vi "GantnerParameters.vi"() -> ()   [LabVIEW 2012]
uses:
  drivers/Gantner/Gantner-Instruments ISMBUS32.llb/ISMBUS_Module.ctl
  drivers/Gantner/Gantner-Instruments ISMBUS32.llb/ISMBUS_Channel.ctl
panel:
  in  "GantnerParameters":T3
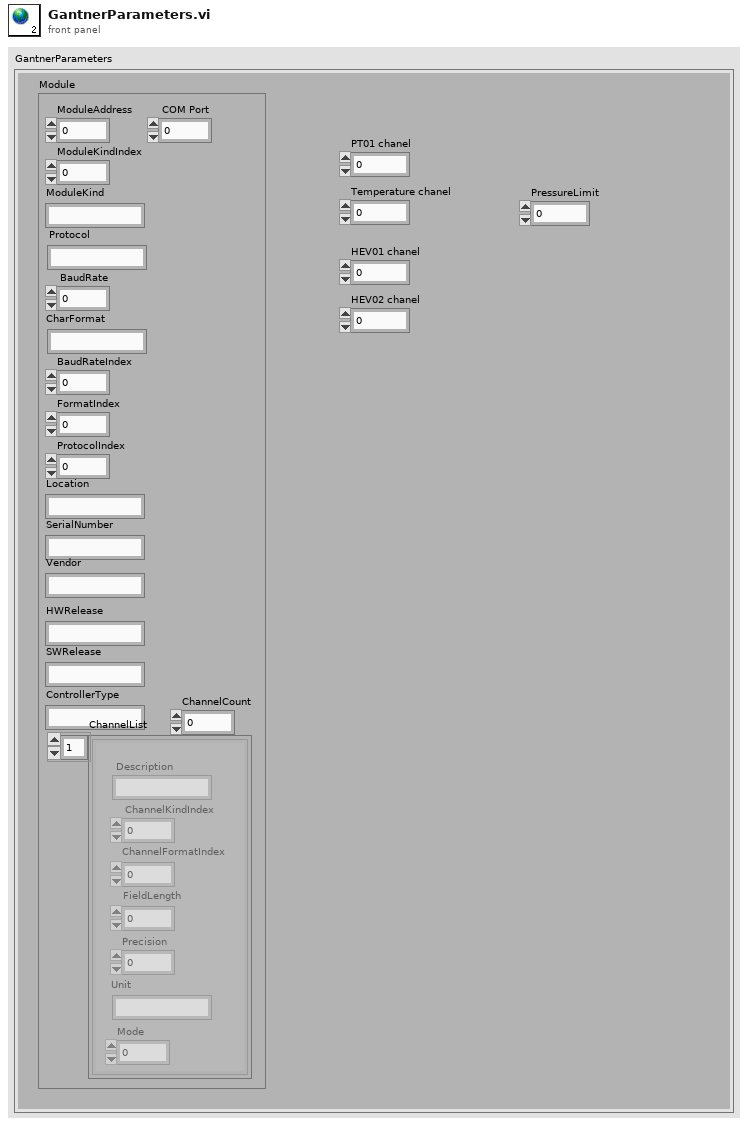
[diagram p1: front panel]
types:
  T1 = typedef "ISMBUS_Module.ctl" = cluster{"ModuleAddress":i32, "ModuleKindIndex":i32, "ModuleKind":string, " Protocol":string, " BaudRate":i32, "CharFormat":string, "BaudRateIndex":i32, "FormatIndex":i32, "ProtocolIndex":i32, "Location":string, "SerialNumber":string, "Vendor":string, "HWRelease":string, "SWRelease":string, "ControllerType":string, "ChannelList":T2[], "ChannelCount":i32, " COM Port":i32}
  T2 = typedef "ISMBUS_Channel.ctl" = cluster{" Description":string, " ChannelKindIndex":i32, "ChannelFormatIndex":i32, " FieldLength":i32, "Precision":i32, "Unit":string, "Mode":i32}
  T3 = cluster{"Module":T1, "PT01 chanel":u32, "Temperature chanel":u32, "HEV01 chanel":u32, "HEV02 chanel":u32, "PressureLimit":dbl}
diagram:
